vi "AadiMakingSwerve - Copy.vi"(0 "X":dbl, 5 "Y":dbl, 7 "Z":dbl) -> (2 "2 power":dbl format="%#_13g", 3 "4 power":dbl format="%#_13g", 4 "1 power":dbl format="%#_13g", 6 "1 angle":dbl format="%#_13g", 8 "2 angle":dbl format="%#_13g", 10 "3 power":dbl format="%#_13g", 14 "4 angle":dbl format="%#_13g", 15 "3 angle":dbl format="%#_13g")   [LabVIEW 2017]
panel:
  out "D":dbl format="%#_13g"
  out "C":dbl format="%#_13g"
  out "B":dbl format="%#_13g"
  out "A":dbl format="%#_13g"
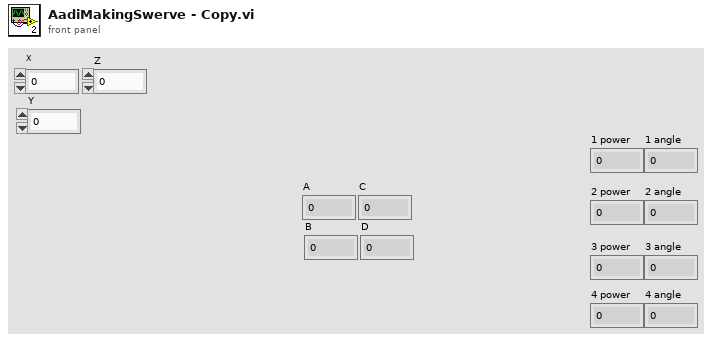
[diagram p1: front panel]
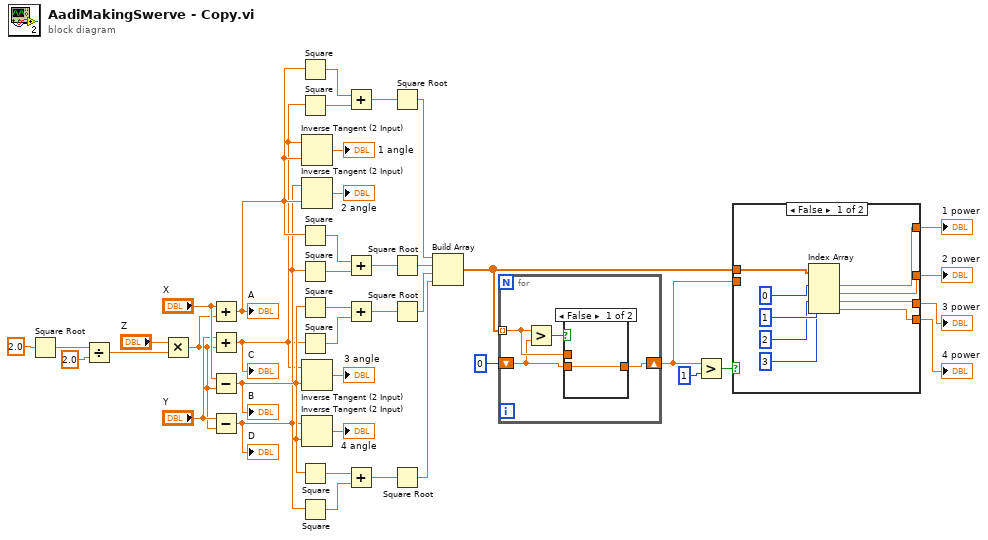
[diagram p0: block diagram]
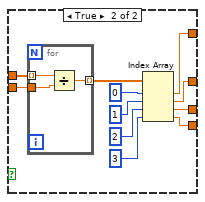
[diagram p2: hidden frame]
diagram:
  n1 = Square Root(x=2.0) -> (sqrt(x)=w40:dbl)
  n2 = Divide(x=w40, y=2.0) -> (x/y=w37:dbl)
  n3 = Multiply(x="Z", y=w37) -> (x*y=w34:dbl)
  n4 = Add(x="X", y=w34) -> (x+y=w17:dbl)
  "A" <- w17
  n5 = Add(x="Y", y=w34) -> (x+y=w14:dbl)
  "C" <- w14
  n6 = Subtract(x="X", y=w34) -> (x-y=w16:dbl)
  "B" <- w16
  n7 = Subtract(x="Y", y=w34) -> (x-y=w15:dbl)
  "D" <- w15
  n8 = Square(x=w17) -> (x^2=w32:dbl)
  n9 = Square(x=w14) -> (x^2=w31:dbl)
  n10 = Square(x=w17) -> (x^2=w27:dbl)
  n11 = Square(x=w15) -> (x^2=w28:dbl)
  n12 = Square(x=w16) -> (x^2=w24:dbl)
  n13 = Square(x=w14) -> (x^2=w23:dbl)
  n14 = Square(x=w16) -> (x^2=w20:dbl)
  n15 = Square(x=w15) -> (x^2=w19:dbl)
  n16 = Inverse Tangent (2 Input)(1:w17, 2:w14) -> (0:→"1 angle":dbl)
  n17 = Inverse Tangent (2 Input)(1:w17, 2:w15) -> (0:→"2 angle":dbl)
  n18 = Inverse Tangent (2 Input)(1:w16, 2:w14) -> (0:→"3 angle":dbl)
  n19 = Inverse Tangent (2 Input)(1:w16, 2:w15) -> (0:→"4 angle":dbl)
  n20 = Add(x=w32, y=w31) -> (x+y=w30:dbl)
  n21 = Add(x=w27, y=w28) -> (x+y=w29:dbl)
  n22 = Add(x=w24, y=w23) -> (x+y=w22:dbl)
  n23 = Add(x=w20, y=w19) -> (x+y=w18:dbl)
  n24 = Square Root(x=w30) -> (sqrt(x)=w7:dbl)
  n25 = Square Root(x=w29) -> (sqrt(x)=w13:dbl)
  n26 = Square Root(x=w22) -> (sqrt(x)=w12:dbl)
  n27 = Square Root(x=w18) -> (sqrt(x)=w11:dbl)
  n28 = Build Array(w7, w13, w12, w11) -> (w6:dbl[])
  n29 = for {
    tunnel: w6 -> [w43] mode=indexing
    shift-right: [w44] -> w5
    shift-left: 0 -> [w42]
    n30 = Greater?(x=w43, y=w42) -> (0:w45:bool)
    n31 = case shown="False" w45 {
      tunnel: [w46 w47] -> w44
      tunnel: w43 -> [_ w47]
      tunnel: w42 -> [w46 _]
      frame False {
      }
      frame True {
      }
    }
  }
  n32 = Greater?(x=w5, y=1) -> (0:w8:bool)
  n33 = case shown="False" w8 {
    tunnel: w6 -> [w56 w67]
    tunnel: w5 -> [_ w66]
    tunnel: [w51 w61] -> w4
    tunnel: [w50 w60] -> w3
    tunnel: [w49 w59] -> w2
    tunnel: [w48 w58] -> w1
    frame False {
      n34 = Index Array(array=w56, index #1=0, index #2=1, index #3=2, index #4=3) -> (element #1=w51:dbl, element #2=w50:dbl, element #3=w49:dbl, element #4=w48:dbl)
    }
    frame True {
      n35 = for {
        tunnel: w67 -> [w70] mode=indexing
        tunnel: w66 -> [w69]
        tunnel: [w68] -> w65 mode=indexing
        n36 = Divide(x=w70, y=w69) -> (x/y=w68:dbl)
      }
      n37 = Index Array(array=w65, index #1=0, index #2=1, index #3=2, index #4=3) -> (element #1=w61:dbl, element #2=w60:dbl, element #3=w59:dbl, element #4=w58:dbl)
    }
  }
  "1 power" <- w4
  "2 power" <- w3
  "3 power" <- w2
  "4 power" <- w1
